vi "TCP-IP Write Data.vi"(5 "Start address":i32, 7 "Data Rigister/Memory":enum16{"Data Register D", "Intiger M"}(ring), 8 "error in (no error)":errorcluster, 9 "M 16 bit Only":bool[](array[boolean]), 10 "Data Write":T1[](array[typedef])=[1, 2, 3], 11 "connection ID":refnum<k5>) -> (0 "error out":errorcluster, 3 "connection ID out":refnum<k5>)   [LabVIEW 2024]
uses:
  Control 100.ctl
panel:
  out "data out":string
  out "bytes to read":i32
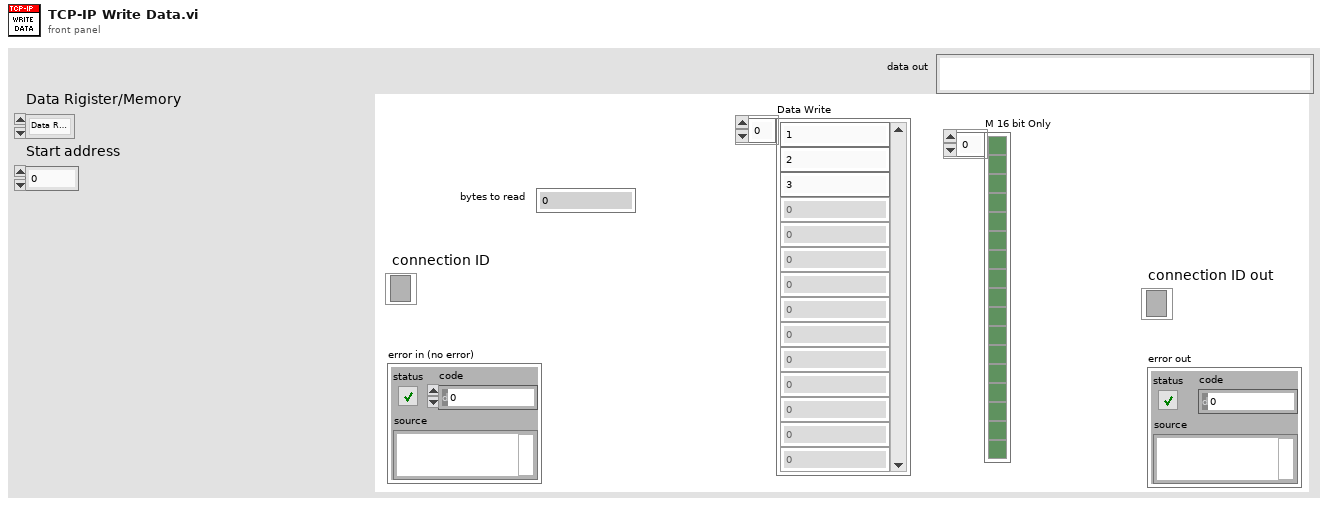
[diagram p1: front panel]
types:
  T1 = typedef "Control 100.ctl" = u16
  T2 = enum16{"Standard", "Buffered", "CRLF", "Immediate"}
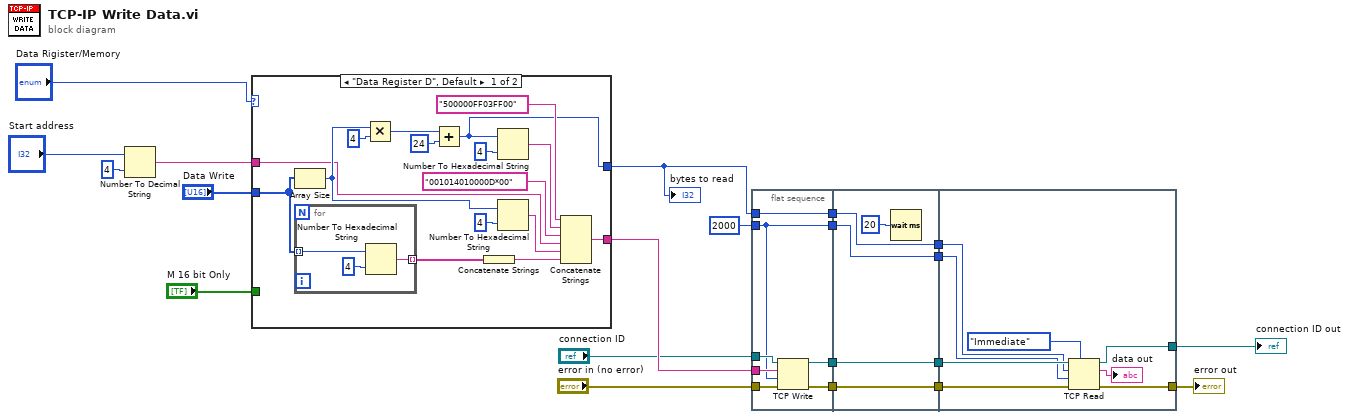
[diagram p0: block diagram]
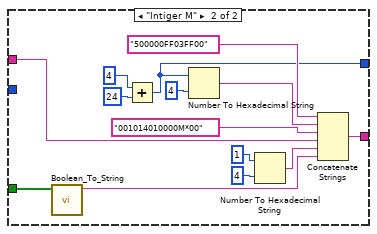
[diagram p2: hidden frame]
diagram:
  n1 = Number To Decimal String(number="Start address", width (-)=i16 4) -> (decimal integer string=w7:string)
  n2 = case shown="\"Data Register D\", Default" "Data Rigister/Memory" {
    tunnel: [w23 w52] -> w4
    tunnel: "M 16 bit Only" -> [_ w51]
    tunnel: w7 -> [w22 w42]
    tunnel: "Data Write" -> [w25 _]
    tunnel: [w24 w41] -> w5
    frame "Data Register D", Default {
      n3 = Array Size(array=w25) -> (size(s)=w33:i32)
      n4 = for {
        tunnel: [w39] -> w34 mode=indexing
        tunnel: w25 -> [w38] mode=indexing
        n5 = Number To Hexadecimal String(1:i16 4 ("width (-)"), 2:w38) -> (0:w39:string)
      }
      n6 = Multiply(x=w33, y=4) -> (x*y=w30:i32)
      n7 = Add(x=w30, y=24) -> (x+y=w24:i32)
      n8 = Concatenate Strings(w34) -> (w36:string)
      n9 = Number To Hexadecimal String(1:i16 4 ("width (-)"), 2:w24) -> (0:w37:string)
      n10 = Number To Hexadecimal String(1:i16 4 ("width (-)"), 2:w33) -> (0:w35:string)
      n11 = Concatenate Strings("500000FF03FF00", w37, "001014010000D*00", w22, w35, w36) -> (w23:string)
    }
    frame "Intiger M" {
      n12 = call "Boolean_To_String.vi"("16 bIT"=w51) -> ("concatenated string 2"=w43:string)  [unwired: 10 in]
      n13 = Add(x=4, y=24) -> (x+y=w41:i32)
      n14 = Number To Hexadecimal String(1:i16 4 ("width (-)"), 2:w41) -> (0:w49:string)
      n15 = Number To Hexadecimal String(1:i16 4 ("width (-)"), 2:1 ("number")) -> (0:w45:string)
      n16 = Concatenate Strings("500000FF03FF00" ("Frame to Read M100 to M107 from FX5U"), w49, "001014010000M*00" ("Frame to Read M100 to M107 from FX5U"), w42, w45, w43) -> (w52:string)
    }
  }
  "bytes to read" <- w5
  n17 = flat-sequence {
    tunnel: w4 -> [w60]
    tunnel: "error in (no error)" -> [w61]
    tunnel: "connection ID" -> [w59]
    tunnel: 2000 ("timeout ms") -> [w56]
    tunnel: [w56] -> w18
    tunnel: [w58] -> w17
    tunnel: [w57] -> w16
    tunnel: [w55] -> w15
    tunnel: w5 -> [w55]
    tunnel: [w66] -> w14
    tunnel: w18 -> [w64]
    tunnel: w17 -> [w66]
    tunnel: [w65] -> w13
    tunnel: w16 -> [w65]
    tunnel: [w64] -> w12
    tunnel: [w63] -> w11
    tunnel: w15 -> [w63]
    tunnel: w14 -> [w72]
    tunnel: w13 -> [w73]
    tunnel: w12 -> [w71]
    tunnel: w11 -> [w69]
    tunnel: [w68] -> w20
    tunnel: [w67] -> w3
    frame #0 {
      n18 = TCP Write(connection ID=w59, data in=w60, error in (no error)=w61, 9:w56) -> (connection ID out=w57:refnum<k5>, error out=w58:errorcluster)  [unwired: 1 out]
    }
    frame #1 {
      n19 = Wait (ms)(milliseconds to wait=u32 20) -> ()  [unwired: 1 out]
    }
    frame #2 {
      n20 = TCP Read(connection ID=w73, bytes to read=w69, error in (no error)=w72, 7:T2."Immediate" ("mode (standard)"), 9:w71) -> (connection ID out=w68:refnum<k5>, data out=→"data out":string, error out=w67:errorcluster)
    }
  }
  "error out" <- w3
  "connection ID out" <- w20
